vi "Assert String Ends With.vi"(5 "Suffix":string, 7 "Message (\"\")":string, 8 "error in (no error)":errorcluster, 10 "String":string) -> (0 "error out":errorcluster)   [LabVIEW 2017, in "Transparent Assertions.lvlib"]
doc: "Asserts that a string ends with the expected suffix. Returns an error if the assertion fails, and optionally appends a custom message to the error."
uses:
  Transparent Assertions.lvlib
  String Ends With/String Ends With.lvclass
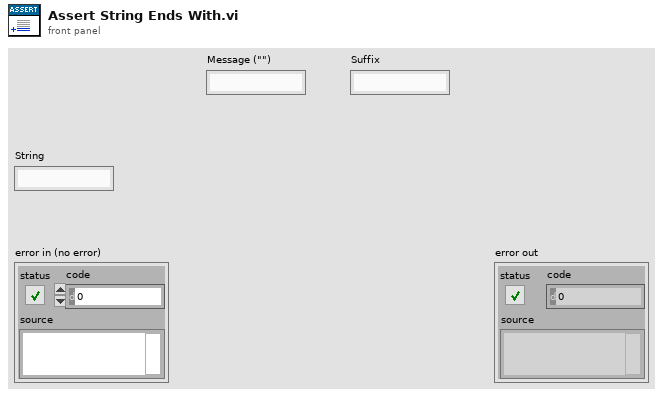
[diagram p1: front panel]
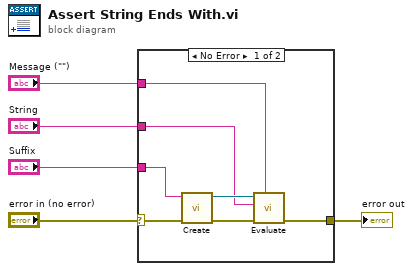
[diagram p0: block diagram]
diagram:
  n1 = case shown="No Error" "error in (no error)" {
    selector: "error in (no error)" -> [w7 w13]
    tunnel: "String" -> [w10 _]
    tunnel: [w9 w13] -> w4
    tunnel: "Message (\"\")" -> [w8 _]
    tunnel: "Suffix" -> [w6 _]
    frame No Error {
      n2 = call "Create.vi"("error in (no error)"=w7, "Suffix"=w6) -> ("error out"=w11:errorcluster, "String Ends With"=w12:refnum<class "String Ends With.lvclass">)  [unwired: 8 in]
      n3 = call-dynamic "Evaluate.vi"("Message (\"\")"=w8, "error in (no error)"=w11, "Actual"=w10, "Constraint in"=w12) -> ("error out"=w9:errorcluster)  [unwired: 6 in, 1 out]
    }
    frame Error {
    }
  }
  "error out" <- w4
